vi "штука.vi"(4 "x0":bool, 5 "x1":bool, 6 "x2":bool, 7 "x3":bool) -> (0 "y0":bool, 1 "y1":bool, 2 "y2":bool, 3 "y3":bool)   [LabVIEW 2013]
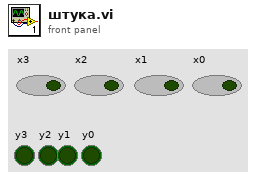
[diagram p1: front panel]
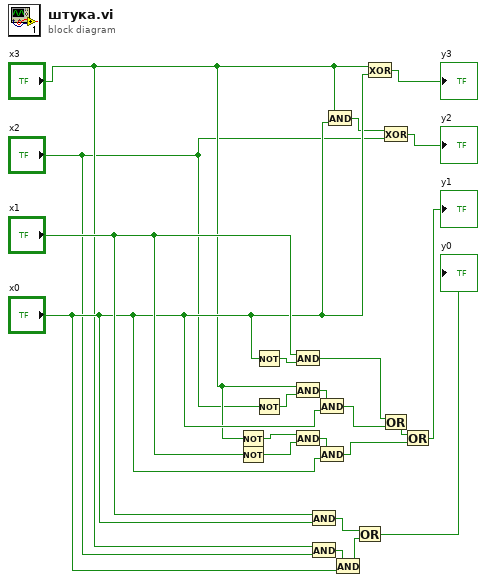
[diagram p0: block diagram]
diagram:
  n1 = Not(x="x3") -> (.not. x?=w12:bool)
  n2 = Not(x="x1") -> (.not. x?=w11:bool)
  n3 = Not(x="x0") -> (.not. x?=w14:bool)
  n4 = Not(x="x2") -> (.not. x?=w13:bool)
  n5 = And(x="x1", y=w14) -> (x .and. y?=w18:bool)
  n6 = And(x="x3", y=w13) -> (x .and. y?=w21:bool)
  n7 = And(x=w12, y=w11) -> (x .and. y?=w20:bool)
  n8 = And(x="x1", y="x0") -> (x .and. y?=w9:bool)
  n9 = And(x="x3", y="x2") -> (x .and. y?=w10:bool)
  n10 = And(x=w21, y="x0") -> (x .and. y?=w17:bool)
  n11 = And(x=w20, y="x0") -> (x .and. y?=w16:bool)
  n12 = And(x="x3", y="x0") -> (x .and. y?=w2:bool)
  n13 = And(x=w10, y="x0") -> (x .and. y?=w8:bool)
  n14 = Or(x=w9, y=w8) -> (x .or. y?=→"y0":bool)
  n15 = Exclusive Or(1:"x0", 2:"x3") -> (0:→"y3":bool)
  n16 = Exclusive Or(1:"x2", 2:w2) -> (0:→"y2":bool)
  n17 = Or(x=w18, y=w17) -> (x .or. y?=w19:bool)
  n18 = Or(x=w19, y=w16) -> (x .or. y?=→"y1":bool)
